vi "自带图像文件读写函数.vi"() -> ()   [LabVIEW 2018]
uses:
  <vilib>/picture/picture.llb/imagedata.ctl
  <vilib>/Analysis/2dsp.llb/2D Convolution (DBL).vi
  <vilib>/picture/picture.llb/Draw True-Color Pixmap.vi
  <vilib>/Analysis/NI_AALPro.lvlib
panel:
  out "error out":errorcluster caption="错误输出"
  out "new picture 3":picture caption="新图片"
  out "new picture 2":picture caption="新图片"
  out "new picture":picture caption="新图片"
  out "image data":T1 caption="图像数据"
  in  "路径":path
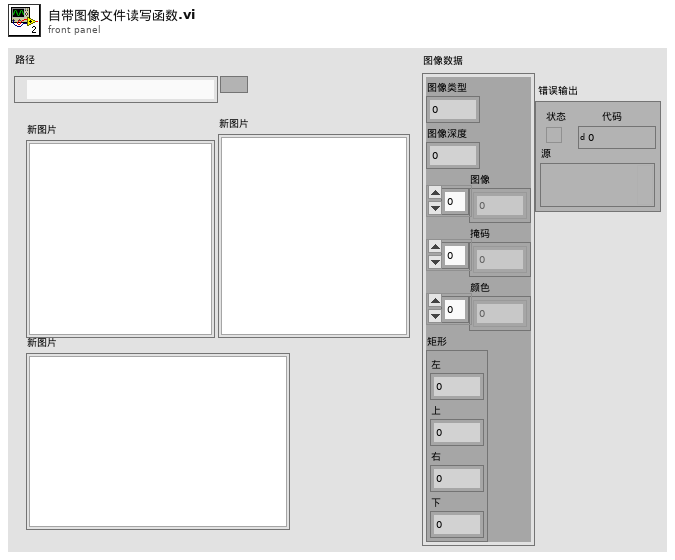
[diagram p1: front panel]
types:
  T1 = typedef "imagedata.ctl" = cluster{"image type":i32, "image depth":i32, "image":u8[], "mask":u8[], "colors":u32[], "Rectangle":cluster{"left":i16, "top":i16, "right":i16, "bottom":i16}}
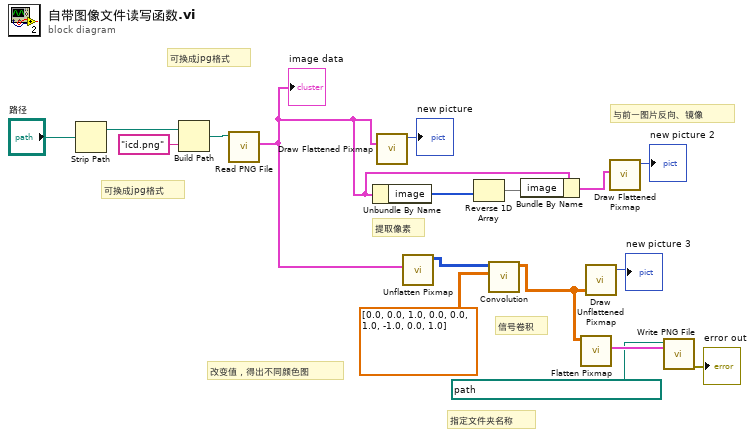
[diagram p0: block diagram]
diagram:
  # "改变值，得出不同颜色图"
  # "指定文件夹名称"
  # "信号卷积"
  # "可换成jpg格式"
  # "可换成jpg格式"
  # "与前一图片反向、镜像"
  # "提取像素"
  n1 = Strip Path(path="路径") -> (stripped path=w16:path)  [unwired: 1 out]
  n2 = Build Path(base path=w16, name or relative path="icd.png" ("名称或相对路径")) -> (appended path=w14:path)
  n3 = call <vilib>:"Read PNG File.vi"("path to PNG file"=w14) -> ("image data"=w8:T1)  [unwired: 8 in, 2 out]
  "image data" <- w8
  n4 = Unbundle By Name(w8) -> ("image"=w12:u8[])
  n5 = call <vilib>:"Draw Flattened Pixmap.vi"("image data"=w8) -> ("new picture"=→"new picture":picture)  [unwired: 8 in]
  n6 = call <vilib>:"Unflatten Pixmap.vi"("image data"=w8) -> ("24-bit pixmap"=w7:u32[][])  [unwired: 4 in, 6 out]
  n7 = Reverse 1D Array(array=w12) -> (reversed array=w11:u8[])
  n8 = call-poly <vilib>:"Convolution.vi"("Y"=dbl[][] [[0.0, 0.0, 1.0], [0.0, 0.0, 1.0], [-1.0, 0.0, 1.0]], "X"=w7) -> ("X * Y"=w4:dbl[][])  [unwired: 8 in, 1 out]
  n9 = Bundle By Name(cluster=w8, "image"=w11) -> (w10:T1)
  n10 = call <vilib>:"Flatten Pixmap.vi"("24-bit pixmap"=w4) -> ("image data"=w3:T1)  [unwired: 10 in]
  n11 = call-poly <vilib>:"Draw Unflattened Pixmap.vi"("data (RGB format)"=w4) -> ("new picture"=→"new picture 3":picture)  [unwired: 8 in]
  n12 = call <vilib>:"Draw Flattened Pixmap.vi"("image data"=w10) -> ("new picture"=→"new picture 2":picture)  [unwired: 8 in]
  n13 = call <vilib>:"Write PNG File.vi"("image data"=w3, "path to PNG file"=path "D:/Labviewprogram/视觉/abc.png") -> ("error out"=→"error out":errorcluster)  [unwired: 8 in, 1 out]
